vi "Minimise.vi"(6 "timeout in ms (-1)":i32=-1, 8 "error in (no error)":errorcluster, 11 "module in":refnum<class "Shell.lvclass">) -> (0 "error out":errorcluster, 3 "module out":refnum<class "Shell.lvclass">, 4 "timed out?":bool)   [LabVIEW 2024, in "Shell.lvclass"]
uses:
  Shell.lvclass
  Shell.lvclass/Shell.ctl
  C:/Git/JA/JQMH/RQMHCore/ModuleCore/Module.lvclass
  C:/Git/JA/JQMH/ModuleTemplates/Shell/Shell.lvclass
  RQMHCore/ModuleCore/Module.lvclass
  RQMHCore/ModuleCore/Reply.ctl
  Minimise Args.ctl
  Minimise ReplyArgs.ctl
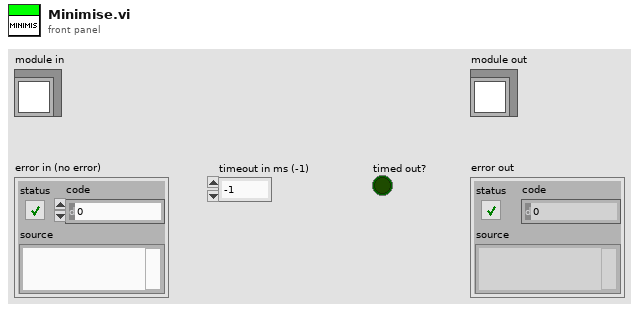
[diagram p1: front panel]
types:
  T1 = typedef "Shell.lvclass/Minimise Args.ctl" = cluster{"null":bool}
  T2 = typedef "Module.lvclass/Reply.ctl" = cluster{"Expects Reply":bool, "Reply":refnum<notifier>}
  T3 = typedef "Shell.lvclass/Minimise ReplyArgs.ctl" = cluster{"null":bool}
  T4 = cluster{"RQMH_REPLYARGS":T3, "error in (no error)":errorcluster}
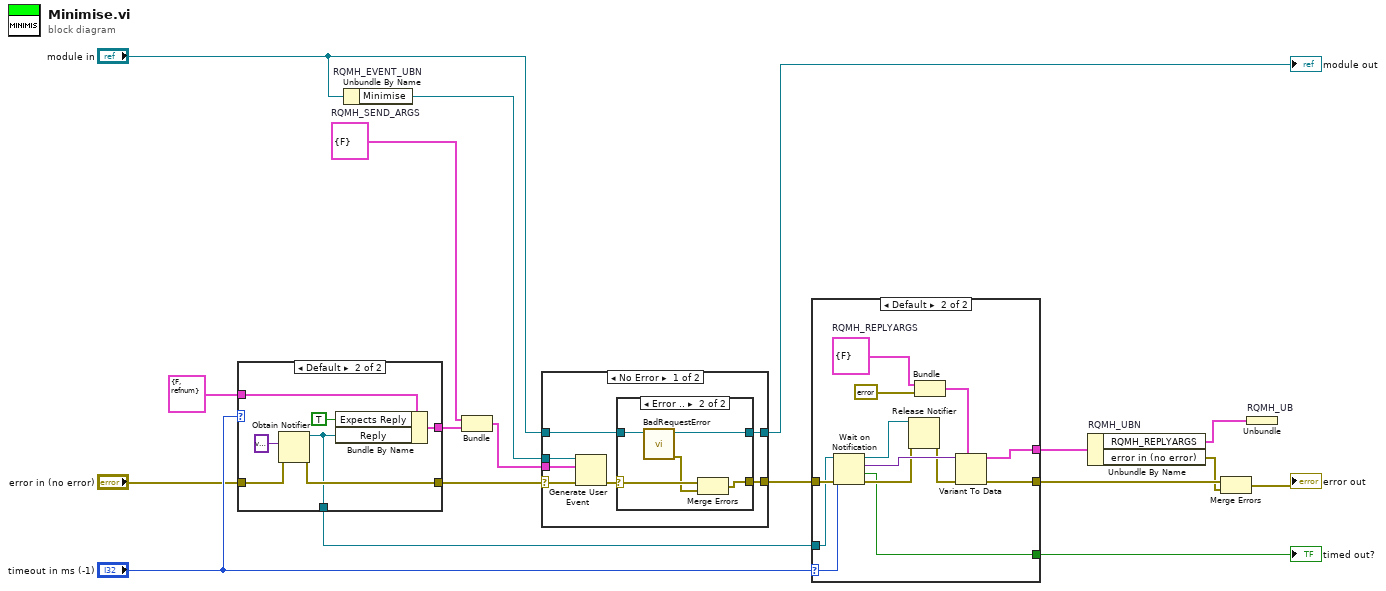
[diagram p0: block diagram]
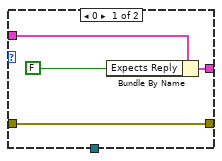
[diagram p4: hidden frame]
diagram:
  w6 = T1 {"null"=FALSE}  # RQMH_SEND_ARGS
  n1 = case shown="Default" "timeout in ms (-1)" {
    tunnel: [w21 w28] -> w18
    tunnel: "error in (no error)" -> [w19 w27]
    tunnel: [w19 w26] -> w16
    tunnel: [_ w25] -> w14
    tunnel: T2 {"Expects Reply"=FALSE, "Reply"=refnum} ("Reply") -> [w22 w24]
    frame 0 {
      n2 = Bundle By Name(cluster=w22, "Expects Reply"=FALSE) -> (w21:T2)
    }
    frame Default {
      n3 = Obtain Notifier(notification data type=variant, error in (no error)=w27) -> (notifier out=w25:refnum<notifier>, error out=w26:errorcluster)  [unwired: 2 in, 1 out]
      n4 = Bundle By Name(cluster=w24, "Expects Reply"=TRUE, "Reply"=w25) -> (w28:T2)
    }
  }
  n5 = Unbundle By Name "RQMH_EVENT_UBN"("module in") -> ("Minimise"=w7:refnum<user-event>)
  n6 = Bundle("RQMH_SEND_ARGS"=w6, "Reply"=w18) -> (w17:cluster{"RQMH_SEND_ARGS":T1, "Reply":T2})  [unwired: 1 in]
  n7 = case shown="No Error" w16 {
    selector: w16 -> [w33 w44]
    tunnel: w17 -> [w36 _]
    tunnel: w7 -> [w35 _]
    tunnel: [w32 w44] -> w15
    tunnel: "module in" -> [w31 w45]
    tunnel: [w30 w45] -> w9
    frame No Error {
      n8 = Generate User Event(user event=w35, event data cluster=w36, error in=w33) -> (error out=w34:errorcluster)  [unwired: 1 in, 1 out]
      n9 = case shown="Error .." w34 {
        selector: w34 -> [w37 w43]
        tunnel: [w37 w42] -> w32
        tunnel: w31 -> [w38 w41]
        tunnel: [w38 w40] -> w30
        frame No Error {
        }
        frame Error {
          n10 = call "BadRequestError.vi"("JQMHModule in"=w41) -> ("error out"=w39:errorcluster, "JQMHModule out"=w40:refnum<class "Shell.lvclass">)  [unwired: 9 in]
          n11 = Merge Errors(w43, w39) -> (w42:errorcluster)
        }
      }
    }
    frame Error {
    }
  }
  "module out" <- w9
  n12 = case shown="Default" "timeout in ms (-1)" {
    selector: "timeout in ms (-1)" -> [_ w50]
    tunnel: w15 -> [w46 w59]
    tunnel: w14 -> [_ w58]
    tunnel: [_ w51] -> w13
    tunnel: [w46 w48] -> w5
    tunnel: [_ w47] -> w4
    frame 0 {
    }
    frame Default {
      w49 = T3 {"null"=FALSE}  # RQMH_REPLYARGS
      n13 = Wait on Notification(notifier=w58, timeout in ms (-1)=w50, error in (no error)=w59) -> (notifier out=w54:refnum<notifier>, notification=w55:variant, timed out?=w51:bool, error out=w53:errorcluster)  [unwired: 1 in]
      n14 = Release Notifier(notifier=w54, error in (no error)=w53) -> (error out=w52:errorcluster)  [unwired: 1 in, 2 out]
      n15 = Bundle("RQMH_REPLYARGS"=w49, "error in (no error)"=errorcluster {"status"=FALSE, "code"=0, "source"=""}) -> (w57:T4)  [unwired: 1 in]
      n16 = Variant To Data(error in=w52, type=w57, Variant=w55) -> (data=w47:T4, error out=w48:errorcluster)
    }
  }
  "timed out?" <- w13
  n17 = Unbundle By Name "RQMH_UBN"(w4) -> ("RQMH_REPLYARGS"=w1:T3, "error in (no error)"=w2:errorcluster)
  n18 = Merge Errors(w5, w2) -> (→"error out":errorcluster)
  n19 = Unbundle "RQMH_UB"(w1) -> ()  [unwired: 1 out]
